vi "Debug.vi"(8 "error in (no error)":errorcluster, 10 "Call Debug":bool, 11 "message":string) -> (0 "error out":errorcluster, 3 "T button?":bool)   [LabVIEW 2024, in "Debug.lvlib"]
uses:
  Debug.lvlib
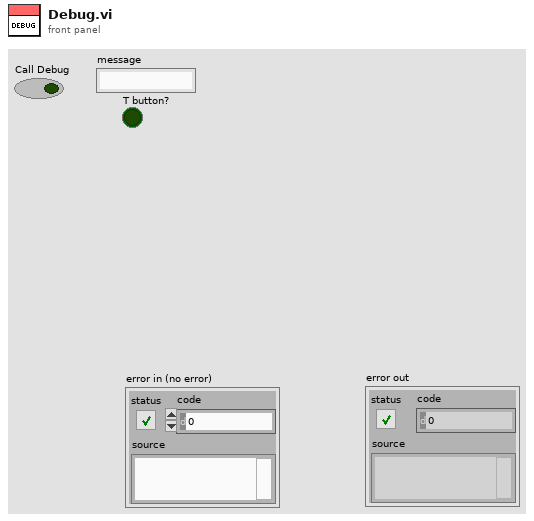
[diagram p1: front panel]
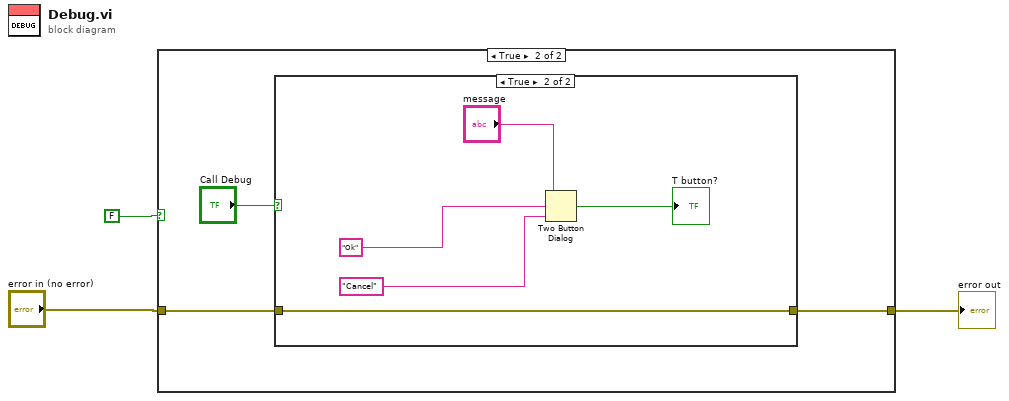
[diagram p0: block diagram]
diagram:
  n1 = case shown="True" FALSE {
    tunnel: "error in (no error)" -> [w4 w6]
    tunnel: [w4 w5] -> w2
    frame False {
    }
    frame True {
      n2 = case shown="True" "Call Debug" {
        tunnel: w6 -> [w8 w9]
        tunnel: [w8 w9] -> w5
        frame False {
        }
        frame True {
          n3 = Two Button Dialog(message="message", 1:"Cancel" ("F button name (\"Cancel\")"), 2:"Ok" ("button name (\"OK\")")) -> (T button?=→"T button?":bool)
        }
      }
    }
  }
  "error out" <- w2
